vi "Save_Histogram.vi"() -> (5 "Plug in titles":string[](array[string]), 7 "Plug in values":string[](array[string]))   [LabVIEW 2010]
uses:
  Controls/Save_Data.ctl
  Globals/Meas_global.vi
  Globals/Plug_in_data_global.vi
  <vilib>/Analysis/NI_AALBase.lvlib
panel:
  out "Waveform Graph":cluster{"Min Value":dbl, dbl, dbl[]}[](graph)
  in  "Data to save":T1(array[cluster])=[{"Ring"=0, "Number of Bins"=50, "Max Value"=0.0, "Min Value"=0.0, "Auto"=TRUE}] {"Ring" items=["Pitot (Uref)", "XW (U)", "XW (V)", "Pitot (Ucrest)", "XW  U1", "XW  U2", "Save Nothing"]}
  in  "Data Type":T2(ring)
  in  "Separation Character":string="\t"
  in  "Precision":i16=2
  in  "Output Directory":path
  in  "File":T3=enum."Save Data"
  # "You must have just these two indicators on the connector pane of the vi"
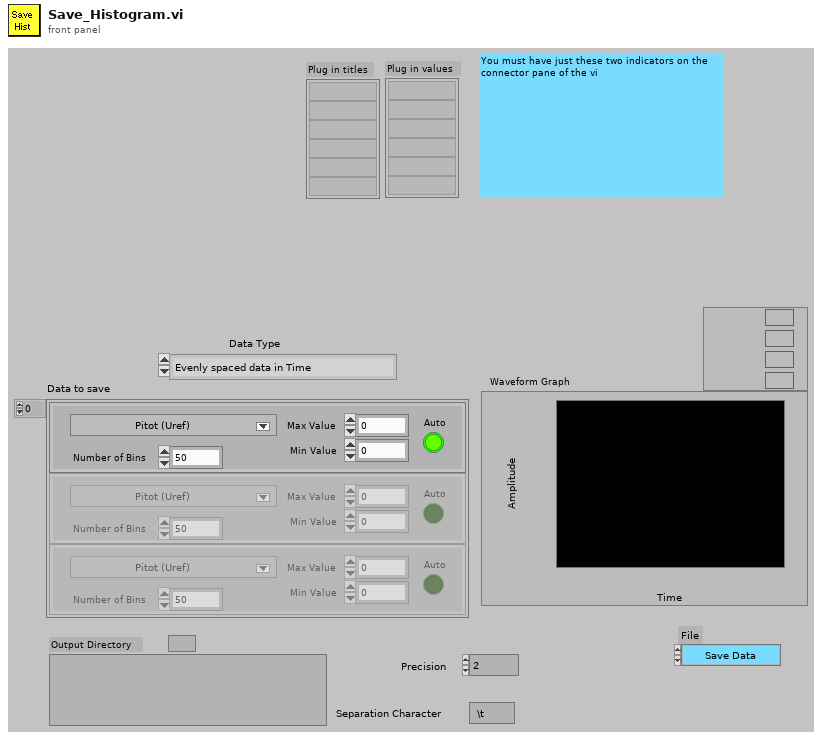
[diagram p1: front panel]
types:
  T1 = cluster{"Ring":i32, "Number of Bins":i32, "Max Value":dbl, "Min Value":dbl, "Auto":bool}[]
  T2 = enum16{"Evenly spaced data in Time", "Unevenly spaced data in Time"}
  T3 = typedef "Save_Data.ctl" = enum16{"Save No Data", "Save Data"}
  T4 = typedef "Analysis_info_cluster.ctl" = cluster{"Colour":u32, "Inst type":T5, "Inst name":string, "Symbol":string, "Code name":string, "Extra Info":string, "Inst Array":T6, "Index":i32, "Voltage Index":i32, "Extra Titles":string[], "Extra Values":string[]}
  T5 = typedef "Inst_type.ctl" = enum16{"Propeller anemometer", "Raw voltage", "Pressure Transducer", "Pitot-static tube", "Preston tube", "Hot wire", "Cross wire 1", "Cross wire 2", "Generic Linear", "Generic Polynomial", "Generic BackPoly", "Fast FID", "Thermocouple", "Cold wire", "Pulsed Wire", "LDA Vel", "LDA Tran time", "LDA Arr time"}
  T6 = typedef "Instrument_Array.ctl" = enum16{"PWA", "LDA", "Analogue"}
  T7 = cluster{"Ring":i32, "Number of Bins":i32, "Max Value":dbl, "Min Value":dbl, "Auto":bool}
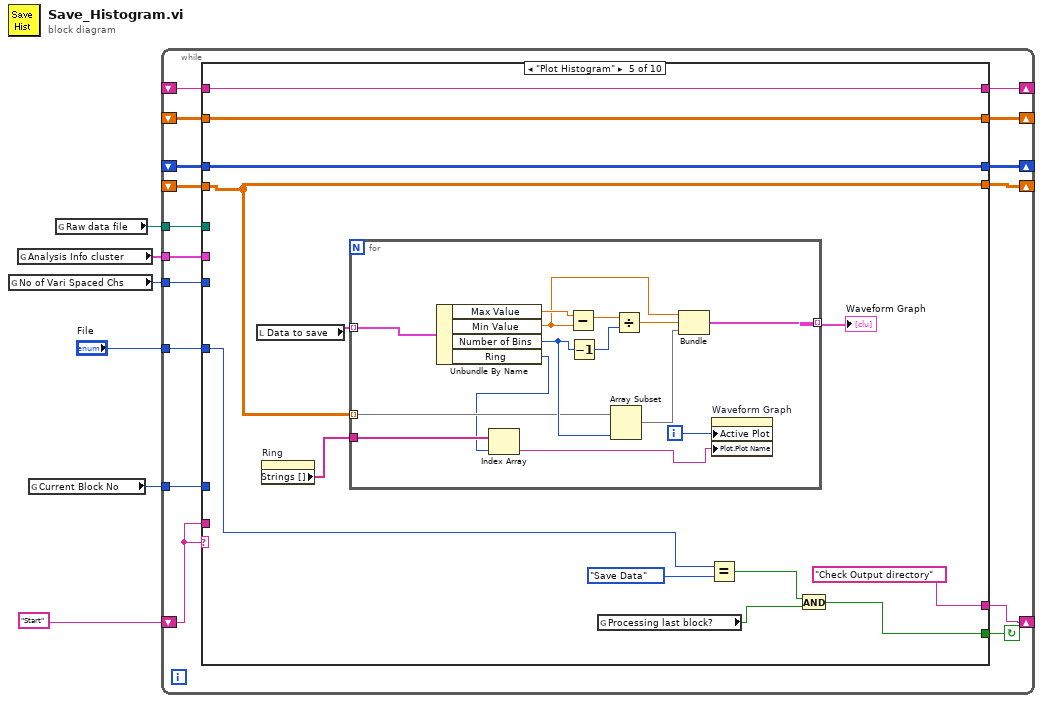
[diagram p0: block diagram]
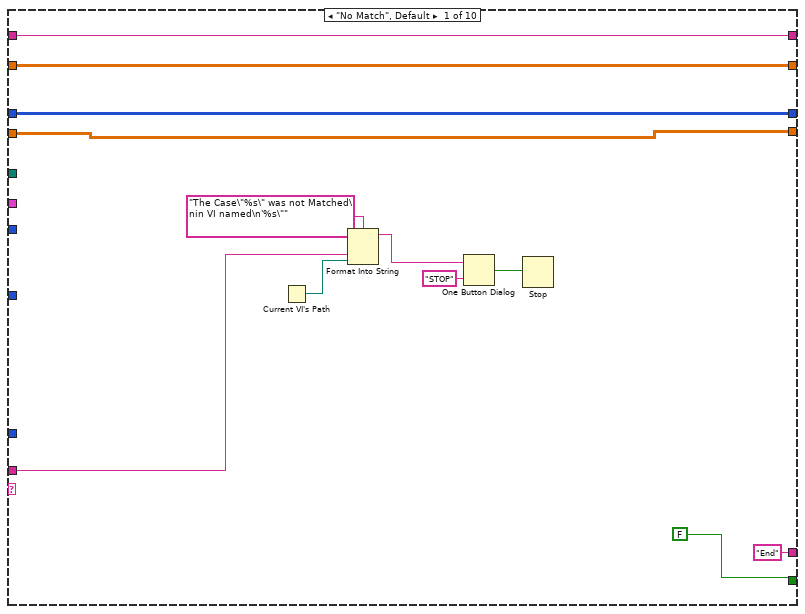
[diagram p2: hidden frame]
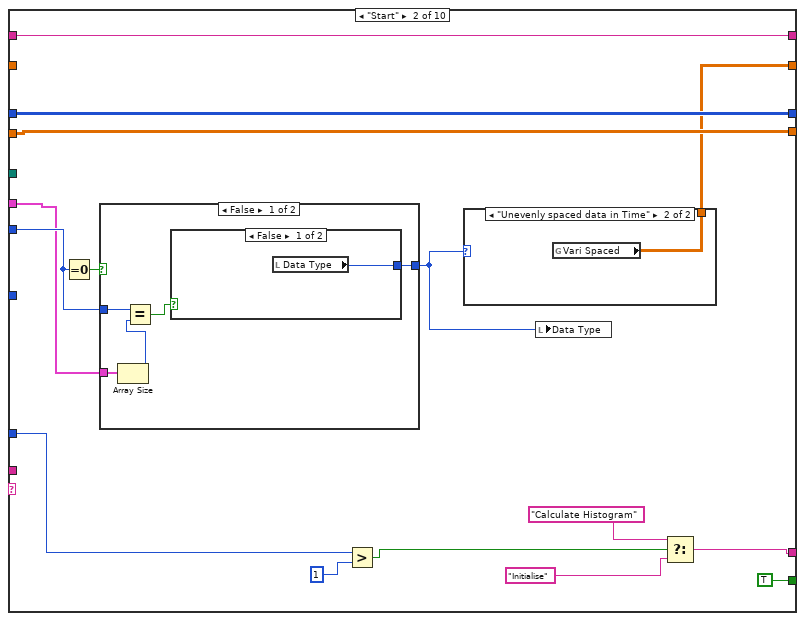
[diagram p3: hidden frame]
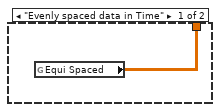
[diagram p4: hidden frame]
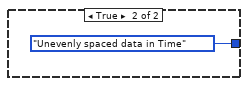
[diagram p5: hidden frame]
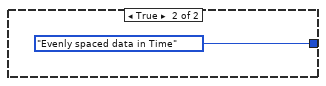
[diagram p6: hidden frame]
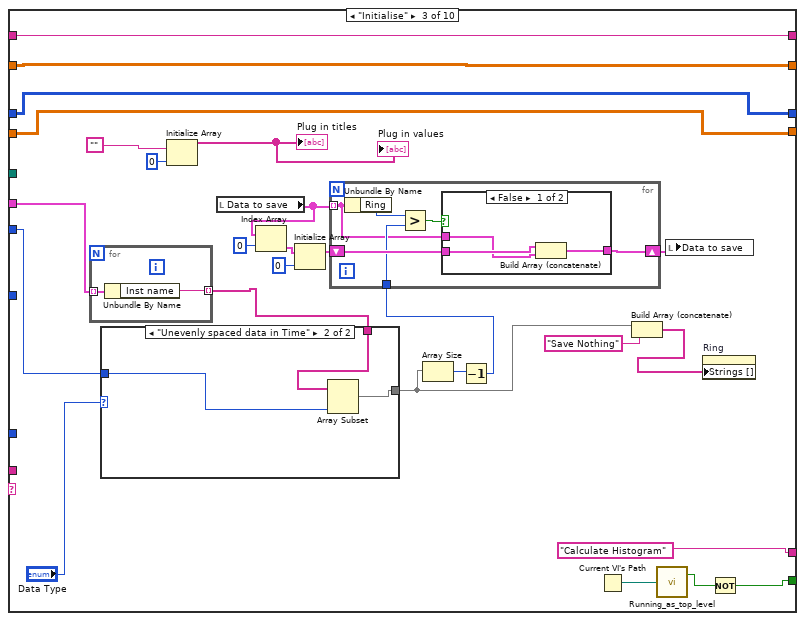
[diagram p7: hidden frame]
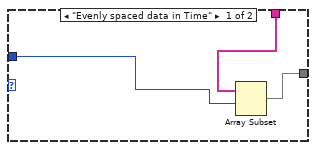
[diagram p8: hidden frame]
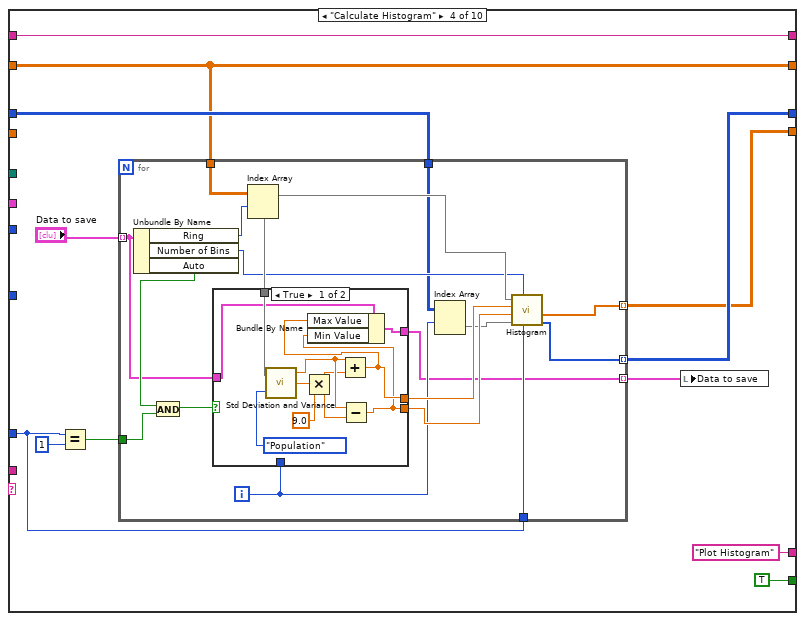
[diagram p10: hidden frame]
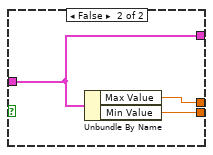
[diagram p11: hidden frame]
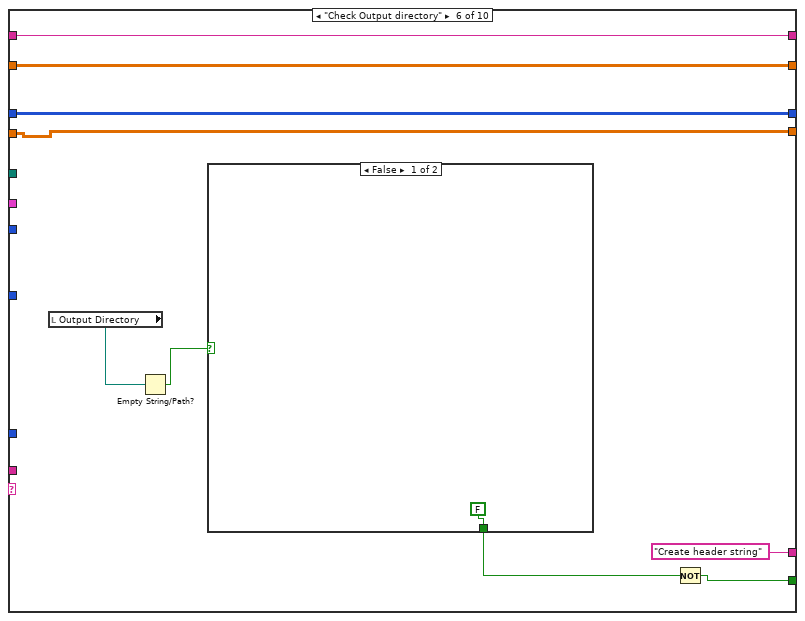
[diagram p12: hidden frame]
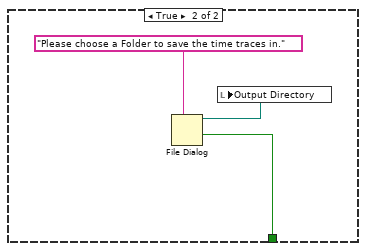
[diagram p13: hidden frame]
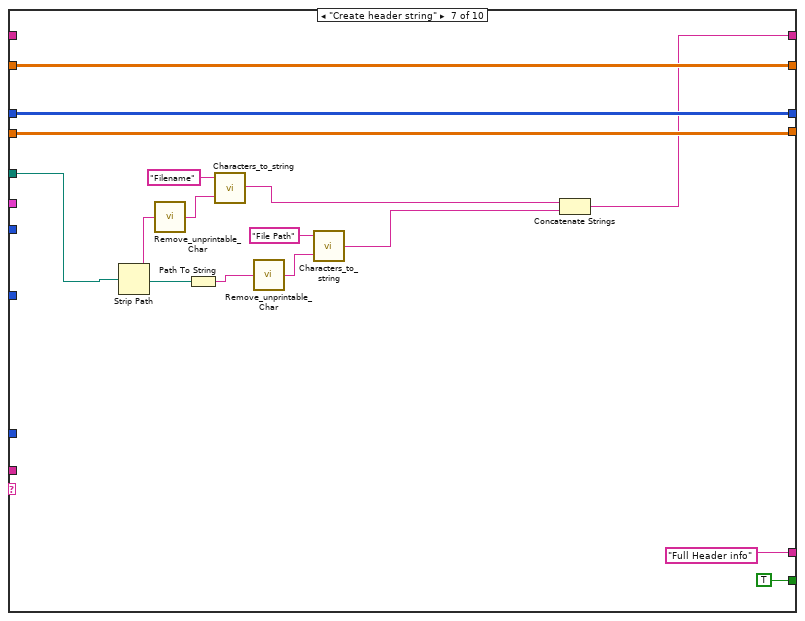
[diagram p14: hidden frame]
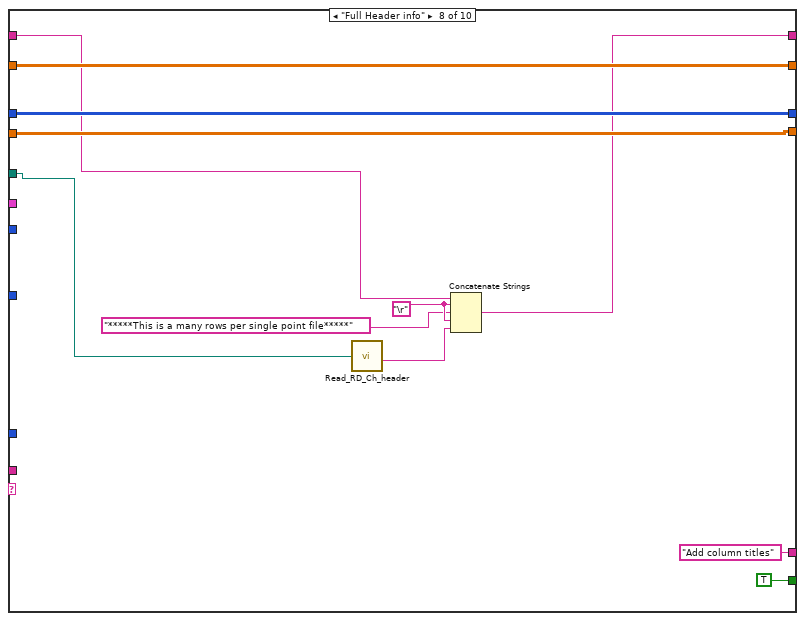
[diagram p15: hidden frame]
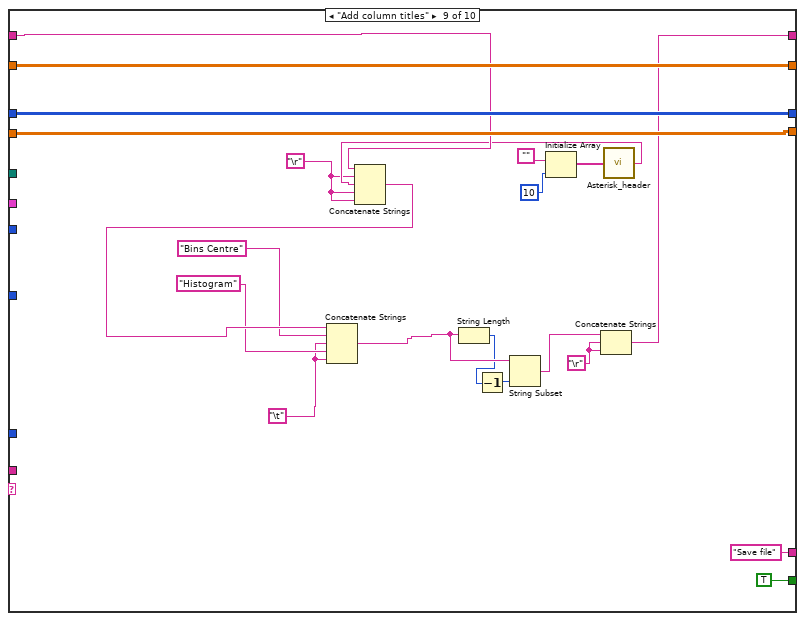
[diagram p16: hidden frame]
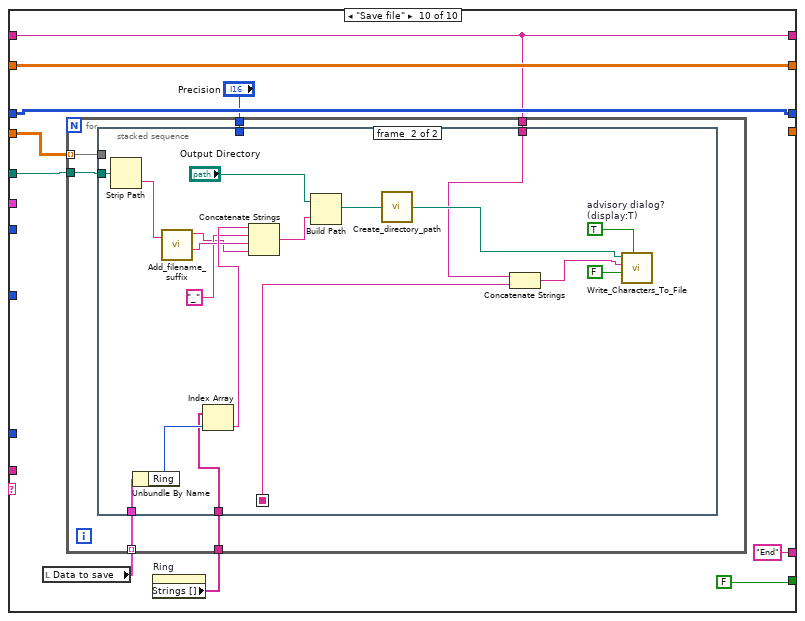
[diagram p17: hidden frame]
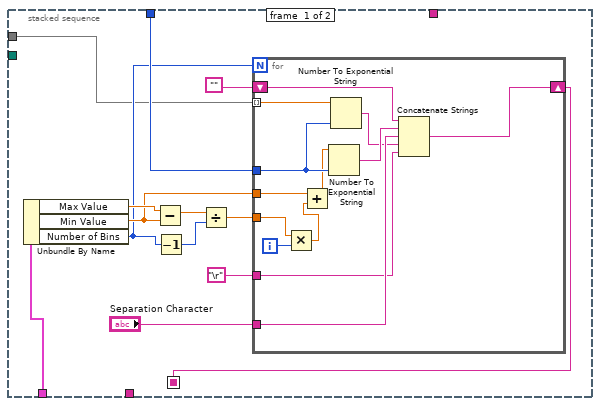
[diagram p18: hidden frame]
diagram:
  n1 = global read "Meas_global.vi" "No of Vari Spaced Chs"() -> (w2:i32)
  n2 = global read "Meas_global.vi" "Analysis Info cluster"() -> (w1:T4[])
  n3 = global read "Meas_global.vi" "Current Block No"() -> (w5:i32)
  n4 = global read "Meas_global.vi" "Raw data file"() -> (w3:path)
  n5 = while {
    shift-left: "Start" -> [w22]
    shift-right: [w21] -> _
    shift-right: [w19] -> _
    shift-left: _ -> [w18]
    shift-right: [w17] -> _
    shift-left: _ -> [w16]
    tunnel: w5 -> [w15]
    tunnel: "File" -> [w14]
    shift-right: [w13] -> _
    shift-left: _ -> [w12]
    tunnel: w3 -> [w11]
    shift-right: [w10] -> _
    shift-left: _ -> [w9]
    tunnel: w2 -> [w8]
    tunnel: w1 -> [w7]
    stop <- w20 continue-if-true
    n6 = case shown="\"Plot Histogram\"" w22 {
      tunnel: ["End" ("t") w44 "Calculate Histogram" ("t") "Plot Histogram" ("t") "Check Output directory" ("t") "Create header string" ("t") "Full Header info" ("t") "Add column titles" ("t") "Save file" ("t") "End" ("t")] -> w21
      tunnel: w22 -> [w30 _ _ _ _ _ _ _ _ _]
      tunnel: [FALSE TRUE w67 TRUE ("Processing last block?") w152 w173 TRUE ("Processing last block?") TRUE ("Processing last block?") TRUE ("Processing last block?") FALSE] -> w20
      tunnel: [w27 w41 w84 w110 w147 w177 w189 w210 w231 _] -> w19
      tunnel: w18 -> [w27 w41 w84 _ w147 w177 w189 w210 w231 w235]
      tunnel: [w26 w43 w60 w111 w149 w179 w190 w211 w232 w242] -> w17
      tunnel: w16 -> [w26 w43 w60 w107 w149 w179 w190 w211 w232 w242]
      tunnel: w15 -> [_ w42 _ w112 _ _ _ _ _ _]
      tunnel: w14 -> [_ _ _ _ w156 _ _ _ _ _]
      tunnel: [w25 w37 w83 w104 w150 w180 w191 w212 w233 w241] -> w13
      tunnel: w12 -> [w25 _ w83 w104 w150 w180 w191 w212 w233 w241]
      tunnel: w11 -> [_ _ _ _ _ _ w192 w203 _ w240]
      tunnel: [w24 w40 w82 w115 w151 w181 w188 w202 w229 w239] -> w10
      tunnel: w9 -> [w24 w40 w82 w115 w151 w181 _ w209 w225 w239]
      tunnel: w8 -> [_ w36 w70 _ _ _ _ _ _ _]
      tunnel: w7 -> [_ w35 w71 _ _ _ _ _ _ _]
      frame "No Match", Default {
        n7 = Current VI's Path() -> (path=w29:path)
        n8 = Format Into String(format string="The Case\"%s\" was not Matched\nin VI named\n'%s\"" ("Format String"), w30, w29) -> (resulting string=w33:string)  [unwired: 2 in, 1 out]
        n9 = One Button Dialog(message=w33, button name ("OK")="STOP") -> (true=w31:bool)
        n10 = Stop(stop? (T)=w31) -> ()
      }
      frame "Start" {
        n11 = Equal To 0?(x=w36) -> (x = 0?=w38:bool)
        n12 = case shown="False" w38 {
          tunnel: [w52 T2."Evenly spaced data in Time" ("Data Type")] -> w39
          tunnel: w35 -> [w56 _]
          tunnel: w36 -> [w54 _]
          frame False {
            n13 = Array Size(array=w56) -> (size(s)=w55:i32)
            n14 = Equal?(x=w54, y=w55) -> (x = y?=w53:bool)
            n15 = case shown="False" w53 {
              tunnel: [w57 T2."Unevenly spaced data in Time" ("Data Type")] -> w52
              frame False {
                n16 = local read "Data Type"() -> (w57:T2)
              }
              frame True {
              }
            }
          }
          frame True {
          }
        }
        n17 = Greater?(x=w42, y=1) -> (0:w46:bool)
        n18 = case shown="\"Unevenly spaced data in Time\"" w39 {
          tunnel: [w50 w51] -> w37
          frame "Evenly spaced data in Time" {
            n19 = global read "Plug_in_data_global.vi" "Equi Spaced"() -> (w50:dbl[][])
          }
          frame "Unevenly spaced data in Time" {
            n20 = global read "Plug_in_data_global.vi" "Vari Spaced"() -> (w51:dbl[][])
          }
        }
        n21 = local write "Data Type"(w39) -> ()
        n22 = Select(t="Calculate Histogram", s=w46, f="Initialise") -> (s? t:f=w44:string)
      }
      frame "Initialise" {
        n23 = for {
          tunnel: w71 -> [w103] mode=indexing
          tunnel: [w102] -> w75 mode=indexing
          n24 = Unbundle By Name(w103) -> ("Inst name"=w102:string)
        }
        n25 = case shown="\"Unevenly spaced data in Time\"" "Data Type" {
          tunnel: w75 -> [w88 w91]
          tunnel: [w87 w90] -> w76
          tunnel: w70 -> [w86 w89]
          frame "Evenly spaced data in Time" {
            n26 = Array Subset(array=w88, index=w86) -> (w87:string[])  [unwired: 1 in]
          }
          frame "Unevenly spaced data in Time" {
            n27 = Array Subset(array=w91, length=w89) -> (w90:string[])  [unwired: 1 in]
          }
        }
        n28 = Initialize Array("", 0) -> (→"Plug in values" →"Plug in titles":string[])
        n29 = local read "Data to save"() -> (w65:T1)
        n30 = Index Array(array=w65, index=0) -> (element=w66:T7)
        n31 = Initialize Array(w66, 0 ("dimension size")) -> (w62:T1)
        n32 = Array Size(array=w76) -> (size(s)=w77:i32)
        n33 = Decrement(x=w77) -> (x-1=w78:i32)
        n34 = for {
          tunnel: w65 -> [w92] mode=indexing
          shift-right: [w95] -> w61
          shift-left: w62 -> [w96]
          tunnel: w78 -> [w94]
          n35 = Unbundle By Name(w92) -> ("Ring"=w93:i32)
          n36 = Greater?(x=w93, y=w94) -> (0:w97:bool)
          n37 = case shown="False" w97 {
            tunnel: w96 -> [w100 w101]
            tunnel: [w99 w101] -> w95
            tunnel: w92 -> [w98 _]
            frame False {
              n38 = Build Array (concatenate)(w100, w98) -> (w99:T1)
            }
            frame True {
            }
          }
        }
        n39 = Current VI's Path() -> (path=w72:path)
        n40 = Build Array (concatenate)(w76, "Save Nothing") -> (w68:string[])
        n41 = call "Running_as_top_level.vi"("Vi path name"=w72) -> ("Top Level"=w73:bool)  [unwired: 1 out]
        n42 = local write "Data to save"(w61) -> ()
        n43 = property on="Ring" class="Ring (strict)"("Strings []"=w68) -> ()  [unwired: 2 in, 2 out]
        n44 = Not(x=w73) -> (.not. x?=w67:bool)
      }
      frame "Calculate Histogram" {
        (unwired) FALSE
        n45 = Equal?(x=w112, y=1) -> (x = y?=w113:bool)
        n46 = for {
          tunnel: [w127] -> w110 mode=indexing
          tunnel: [w132] -> w111 mode=indexing
          tunnel: w104 -> [w126]
          tunnel: "Data to save" -> [w120] mode=indexing
          tunnel: w113 -> [w123]
          tunnel: w112 -> [w119]
          tunnel: w107 -> [w118]
          tunnel: [w117] -> w109 mode=indexing
          i -> [w128]
          n47 = Unbundle By Name(w120) -> ("Ring"=w125:i32, "Number of Bins"=w124:i32, "Auto"=w122:bool)
          n48 = And(x=w122, y=w123) -> (x .and. y?=w121:bool)
          n49 = Index Array(array=w126, index (row)=w125) -> (element=w129:dbl[])  [unwired: 1 in]
          n50 = case shown="True" w121 {
            tunnel: [w135 w145] -> w131
            tunnel: [w134 w144] -> w130
            tunnel: w128 -> [_ _]
            tunnel: w129 -> [w142 _]
            tunnel: w120 -> [w136 w143]
            tunnel: [w133 w143] -> w117
            frame True {
              n51 = call <vilib>:"Std Deviation and Variance.vi"("X"=w142, "Weighting (Sample)"=enum16{"Sample", "Population"}."Population") -> ("mean"=w141:dbl, "standard deviation"=w140:dbl)  [unwired: 1 out]
              n52 = Multiply(x=w140, y=9.0) -> (x*y=w138:dbl)
              n53 = Add(x=w141, y=w138) -> (x+y=w135:dbl)
              n54 = Subtract(x=w141, y=w138) -> (x-y=w134:dbl)
              n55 = Bundle By Name(cluster=w136, "Max Value"=w135, "Min Value"=w134) -> (w133:T7)
            }
            frame False {
              n56 = Unbundle By Name(w143) -> ("Max Value"=w145:dbl, "Min Value"=w144:dbl)
            }
          }
          n57 = Index Array(array=w118, index (row)=w128) -> (element=w116:i32[])  [unwired: 1 in]
          n58 = call "Histogram.vi"("Current Block No"=w119, "No of bins"=w124, "Shift Hist"=w116, "Min value"=w130, "Max value"=w131, "X"=w129) -> ("Shift Hist"=w132:i32[], "Histogram of X"=w127:dbl[])  [unwired: 1 in, 2 out]
        }
        n59 = local write "Data to save"(w109) -> ()
      }
      frame "Plot Histogram" {
        n60 = local read "Data to save"() -> (w158:T1)
        n61 = property on="Ring" class="Ring (strict)"() -> ("Strings []"=w146:string[])  [unwired: 2 in, 2 out]
        n62 = for {
          tunnel: w158 -> [w169] mode=indexing
          tunnel: w147 -> [w165] mode=indexing
          tunnel: [w163] -> w157 mode=indexing
          tunnel: w146 -> [w161]
          i -> [w162]
          n63 = Unbundle By Name(w169) -> ("Max Value"=w172:dbl, "Min Value"=w167:dbl, "Number of Bins"=w166:i32, "Ring"=w160:i32)
          n64 = Index Array(array=w161, index=w160) -> (element=w159:string)
          n65 = Subtract(x=w172, y=w167) -> (x-y=w171:dbl)
          n66 = Decrement(x=w166) -> (x-1=w170:i32)
          n67 = Array Subset(array=w165, length=w166) -> (w164:dbl[])  [unwired: 1 in]
          n68 = Divide(x=w171, y=w170) -> (x/y=w168:dbl)
          n69 = Bundle("Min Value"=w167, w168, w164) -> (w163:cluster{"Min Value":dbl, dbl, dbl[]})  [unwired: 1 out]
          n70 = property on="Waveform Graph" class="WFGraph (strict)"("Active Plot"=w162, "Plot.Plot Name"=w159) -> ()  [unwired: 2 in, 2 out]
        }
        "Waveform Graph" <- w157
        n71 = global read "Meas_global.vi" "Processing last block?"() -> (w155:bool)
        n72 = Equal?(x=w156, y=Save_Data."Save Data" ("File")) -> (x = y?=w153:bool)
        n73 = And(x=w153, y=w155) -> (x .and. y?=w152:bool)
      }
      frame "Check Output directory" {
        n74 = local read "Output Directory"() -> (w175:path)
        n75 = Empty String/Path?(string/path=w175) -> (empty?=w176:bool)
        n76 = case shown="False" w176 {
          tunnel: [FALSE ("cancelled") w183] -> w174
          frame False {
          }
          frame True {
            n77 = File Dialog(7:"Please choose a Folder to save the time traces in." ("prompt")) -> (1:w183:bool, 3:w185:path)  [unwired: 1 in, 7 out]
            n78 = local write "Output Directory"(w185) -> ()
          }
        }
        n79 = Not(x=w174) -> (.not. x?=w173:bool)
      }
      frame "Create header string" {
        n80 = Strip Path(path=w192) -> (stripped path=w196:path, name=w200:string)
        n81 = call "Remove_unprintable_Char.vi"("Input String"=w200) -> ("Output String"=w199:string)
        n82 = Path To String(path=w196) -> (string=w195:string)
        n83 = call "Characters_to_string.vi"("Characters to write"=w199, "Label for characters"="Filename") -> ("Output string"=w194:string)
        n84 = call "Remove_unprintable_Char.vi"("Input String"=w195) -> ("Output String"=w198:string)
        n85 = call "Characters_to_string.vi"("Characters to write"=w198, "Label for characters"="File Path") -> ("Output string"=w193:string)
        n86 = Concatenate Strings(w194, w193) -> (w188:string)
      }
      frame "Full Header info" {
        w206 = "\r"
        n87 = call "Read_RD_Ch_header.vi"("Raw data file"=w203) -> ("Ch string"=w204:string)  [unwired: 3 out]
        n88 = Concatenate Strings(w209, w206, "*****This is a many rows per single point file*****", w206, w204) -> (w202:string)
      }
      frame "Add column titles" {
        w213 = "\t"
        w219 = "\r"
        w220 = "\r"
        n89 = Initialize Array("", 10) -> (w224:string[])
        n90 = call "Asterisk_header.vi"("Channel names"=w224) -> ("Header string"=w221:string)
        n91 = Concatenate Strings(w225, w219, w221, w219, w219) -> (w230:string)
        n92 = Concatenate Strings(w230, "Bins Centre", w213, "Histogram", w213) -> (w218:string)
        n93 = String Length(string=w218) -> (length=w215:i32)
        n94 = Decrement(x=w215) -> (x-1=w216:i32)
        n95 = String Subset(string=w218, length (rest)=w216) -> (substring=w217:string)  [unwired: 1 out]
        n96 = Concatenate Strings(w217, w220, w220) -> (w229:string)
      }
      frame "Save file" {
        n97 = local read "Data to save"() -> (w237:T1)
        n98 = property on="Ring" class="Ring (strict)"() -> ("Strings []"=w234:string[])  [unwired: 2 in, 2 out]
        n99 = for {
          tunnel: w240 -> [w249]
          tunnel: w239 -> [w248]
          tunnel: w237 -> [w247] mode=indexing
          tunnel: "Precision" -> [w246]
          tunnel: w235 -> [w245] mode=indexing
          tunnel: w234 -> [w244]
          n100 = stacked-sequence {
            seq-local: [w251 _] -> [_ w287]
            tunnel: w249 -> [_ w293]
            tunnel: w248 -> [_ w288]
            tunnel: w247 -> [w262 w285]
            tunnel: w246 -> [w258 _]
            tunnel: w245 -> [w254 _]
            tunnel: w244 -> [_ w283]
            frame #0 {
              n101 = Unbundle By Name(w262) -> ("Max Value"=w261:dbl, "Min Value"=w256:dbl, "Number of Bins"=w255:i32)
              n102 = Subtract(x=w261, y=w256) -> (x-y=w260:dbl)
              n103 = Decrement(x=w255) -> (x-1=w259:i32)
              n104 = Divide(x=w260, y=w259) -> (x/y=w257:dbl)
              n105 = for {
                N: w255 -> [_]
                tunnel: w258 -> [w270]
                tunnel: w257 -> [w274]
                tunnel: w256 -> [w272]
                tunnel: w254 -> [w271] mode=indexing
                tunnel: "Separation Character" -> [w267]
                shift-right: [w264] -> w251
                shift-left: "" -> [w265]
                tunnel: "\r" -> [w263]
                i -> [w275]
                n106 = Multiply(x=w274, y=w275) -> (x*y=w273:dbl)
                n107 = Add(x=w272, y=w273) -> (x+y=w269:dbl)
                n108 = Number To Exponential String(number=w269, precision (6)=w270) -> (E-format string=w268:string)  [unwired: 2 out]
                n109 = Number To Exponential String(number=w271, precision (6)=w270) -> (E-format string=w266:string)  [unwired: 2 out]
                n110 = Concatenate Strings(w265, w268, w267, w266, w263) -> (w264:string)
              }
            }
            frame #1 {
              w290 = TRUE  # advisory dialog? (display:T)
              n111 = Strip Path(path=w293) -> (name=w282:string)  [unwired: 1 out]
              n112 = Unbundle By Name(w285) -> ("Ring"=w284:i32)
              n113 = call "Add_filename_suffix.vi"("Filename"=w282) -> ("Original Suffix"=w278:string, "Base name"=w280:string)  [unwired: 1 in, 2 out]
              n114 = Index Array(array=w283, index=w284) -> (element=w281:string)
              n115 = Concatenate Strings(w281, "_" ("string"), w280, w278) -> (w277:string)
              n116 = Build Path(base path="Output Directory", name or relative path=w277) -> (appended path=w292:path)
              n117 = call "Create_directory_path.vi"("Path name"=w292) -> ("Path name Out"=w291:path)
              n118 = Concatenate Strings(w288, w287) -> (w286:string)
              n119 = call "Write_Characters_To_File.vi"("file path (dialog if empty)"=w291, "advisory dialog? (display:T)"=w290, "character string"=w286, "append to file? (new file:F)"=FALSE) -> ()  [unwired: 1 in, 4 out]
            }
          }
        }
      }
    }
  }
